vi "Decode Chunk (subVI).vi"(8 "error in (no error)":errorcluster, 10 "Chunk (without size)":string) -> (0 "error out":errorcluster, 1 "Checksum Failed?":bool, 2 "Flattened Data":u8[](array[numeric]))   [LabVIEW 2015]
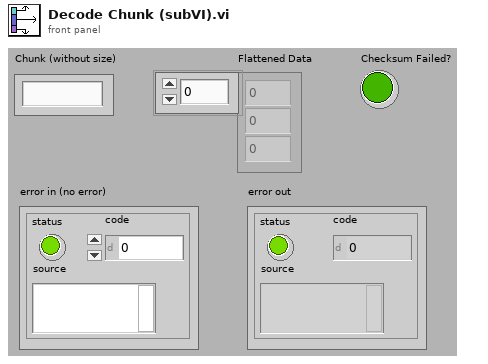
[diagram p1: front panel]
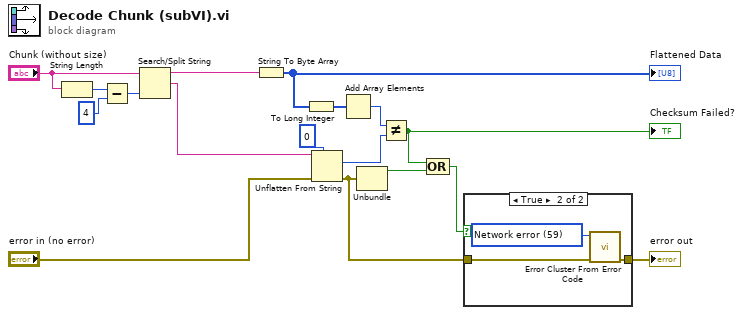
[diagram p0: block diagram]
diagram:
  n1 = String Length(string="Chunk (without size)") -> (length=w15:i32)
  n2 = Subtract(x=w15, y=4) -> (x-y=w13:i32)
  n3 = Search/Split String(string="Chunk (without size)", offset (0)=w13) -> (substring before match=w4:string, match + rest of string=w11:string)  [unwired: 2 out]
  n4 = String To Byte Array(string=w4) -> (unsigned byte array=w3:u8[])
  "Flattened Data" <- w3
  n5 = To Long Integer(number=w3) -> (32bit integer=w17:i32[])
  n6 = Unflatten From String(type=0 ("y"), binary string=w11, error in (no error)="error in (no error)") -> (value=w9:i32, error out=w1:errorcluster)  [unwired: 3 out]
  n7 = Add Array Elements(numeric array=w17) -> (sum=w10:i32)
  n8 = Unbundle(w1) -> ("status"=w7:bool)  [unwired: 2 out]
  n9 = Not Equal?(x=w10, y=w9) -> (x != y?=w5:bool)
  "Checksum Failed?" <- w5
  n10 = Compound Arithmetic op=OR(w5, w7) -> (w6:bool)
  n11 = case shown="True" w6 {
    tunnel: w1 -> [w18 w21]
    tunnel: [w18 w20] -> w8
    frame False {
    }
    frame True {
      w19 = 59 items=["No error", "Argument error", "Memory is full", "Out of zone", "End of file", "File already open", "Generic file I/O error", "File not found", "File permission error", "Disk is full", "Duplicate path", "Too many files open", "System feature not enabled", "Resource file not found", "Cannot add resource", "Resource not found", "Image not found", "Image memory error", "Pen does not exist", "Config type invalid", "Config token not found", "Config parse error", "Config memory error", "Bad external code format", "Bad external code offset", "External code not present", "Null window", "Destroy window error", "Null menu", "Print aborted", "Bad print record", "Print driver error", "Windows error during printing", "Memory error during printing", "Print dialog error", "Generic print error", "Invalid device refnum", "Device not found", "Device parameter error", "Device unit error", "Cannot open device", "Device call aborted", "Generic error", "Cancelled by user", "Object ID too low", "Object ID too high", "Object not in heap", "Unknown heap", "Unknown object (invalid DefProc)", "Unknown object (DefProc not in table)", "Message out of range", "Invalid (null) method", "Unknown message", "Manager call not supported", "Bad address", "Network operation in progress", "Network operation timed out", "Connection is busy", "Network attribute not supported", "Network error", "Address in use", "System out of memory", "Connection aborted", "Connection refused", "Not connected", "Already connected", "Connection closed", "Initialization error (interapplication manager)", "Bad occurrence", "Wait on unbound occurrence handler", "Occurrence queue overflow", "Datalog type conflict", "Unused", "Unrecognized type (interapplication manager)", "Memory corrupt", "Failed to make temporary DLL", "Old CIN version", "Drag socket not found", "Failed to load drop-object", "Failed to register OLE object", "Failed to release OLE object", "Format specifier type mismatch", "Unknown format specifier", "Too few format specifiers", "Too many format specifiers", "Scan failed", "Newer CIN version", "Error converting to variant", "Runtime menu error", "Password tampered", "Variant attribute not found", "Incompatible variant data type", "Event data is not available", "Event Store is not present", "Occurrence is not found", "Event Queue is not created", "Event info is not available in the type library", "Refnum passed is NULL", "Error retrieving Class GUID", "Error retrieving CoClass GUID", "Error retrieving TypeLib GUID.", "Bad built application magic bytes.", "Specific driver is different from the specific driver associated with the Logical Name.", "There is no session opened to the class driver.", "Max Error", "MAX - Error with config objects", "MAX - Error loading configuration", "MAX - Group not supported", "Singlecast connections can not send to multicast addresses.", "Multicast connections can not send to singlecast addresses.", "Specified IP address not in multicast address range.", "Attempt to write to read-only multicast connection.", "Attempt to read from write-only multicast connection.", "The buffer used to receive a datagram was smaller than the datagram itself"]
      n12 = call <vilib>:"Error Cluster From Error Code.vi"("error in (no error)"=w21, "error code (0)"=w19) -> ("error out"=w20:errorcluster)  [unwired: 1 in, 6 out]
    }
  }
  "error out" <- w8
